vi "读取excel.vi"(10 "Worksheets":i32=1, 11 "Filename":string) -> (3 "数据":string[][](array[string]))   [LabVIEW 2020]
panel:
  in  "Excel._Application":refnum<k7>
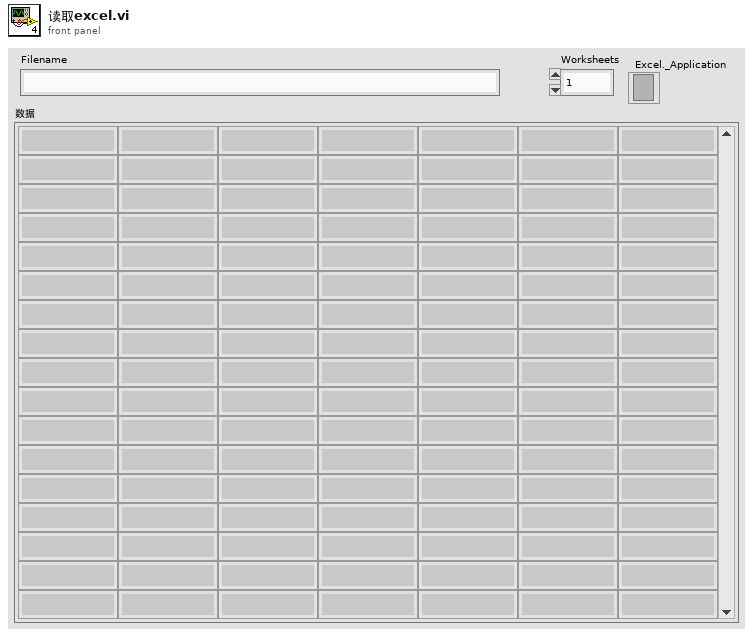
[diagram p1: front panel]
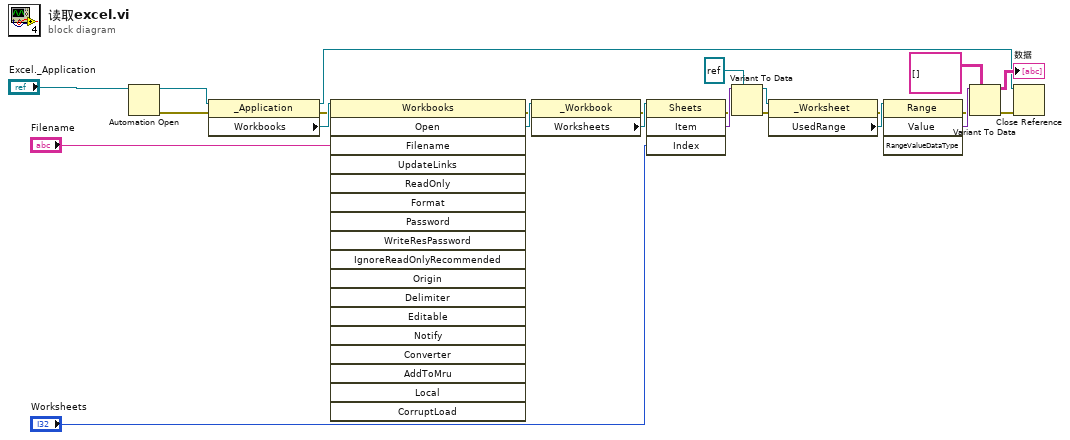
[diagram p0: block diagram]
diagram:
  n1 = Automation Open(Automation Refnum="Excel._Application") -> (Automation Refnum=w1:refnum<k7>, error out=w11:errorcluster)  [unwired: 3 in]
  n2 = property class="_Application"(reference=w1, error in=w11) -> (reference out=w3:refnum<k7>, error out=w10:errorcluster, "Workbooks"=w23:refnum<k7>)
  n3 = invoke class="Workbooks" method="Open"(reference=w23, error in=w10, "Filename"="Filename") -> (error out=w9:errorcluster, "Open"=w21:refnum<k7>)  [unwired: 15 in, 16 out]
  n4 = property class="_Workbook"(reference=w21, error in=w9) -> (error out=w19:errorcluster, "Worksheets"=w20:refnum<k7>)  [unwired: 1 out]
  n5 = invoke class="Sheets" method="Item"(reference=w20, error in=w19, "Index"="Worksheets") -> (error out=w8:errorcluster, "Item"=w17:variant)  [unwired: 1 in, 2 out]
  n6 = Variant To Data(error in=w8, type=refnum<k7> refnum ("Excel._Worksheet"), Variant=w17) -> (data=w15:refnum<k7>, error out=w7:errorcluster)
  n7 = property class="_Worksheet"(reference=w15, error in=w7) -> (error out=w6:errorcluster, "UsedRange"=w14:refnum<k7>)  [unwired: 1 out]
  n8 = invoke class="Range" method="Value"(reference=w14, error in=w6) -> (error out=w5:errorcluster, "Value"=w13:variant)  [unwired: 2 in, 2 out]
  n9 = Variant To Data(error in=w5, type=string[][] [], Variant=w13) -> (data=→"数据":string[][], error out=w2:errorcluster)
  n10 = Close Reference(reference=w3, error in (no error)=w2) -> ()  [unwired: 1 out]
